vi "R4SetOtherConstants.vi"(6 "cRIONo":i32=1, 7 "LabVIEW Web Service Request":refnum<class "Web Request.lvclass">, 8 "ReactorNo":i32=1, 9 "Value":string, 10 "Constant":string, 11 "Write":bool) -> (1 "NewValue":string, 2 "OldValue":string, 3 "Status":string)   [LabVIEW 2016]
uses:
  <vilib>/wsapi/Web Request.lvclass
  <resource>/objmgr/ni.var.rc
panel:
  in  "LabVIEW Web Service Request 2":refnum<class "Web Request.lvclass">
  # "Use the Web Service Request input terminal to call the VIs on the Web Services palette. Do not remove it from the connector pane unless you don't need access to the palette."
  # "Each additional control wired to the connector pane will be available as an input in the URL. To include an indicator in terminal-mode output (the default setting), it must also be wired to the connector pane."
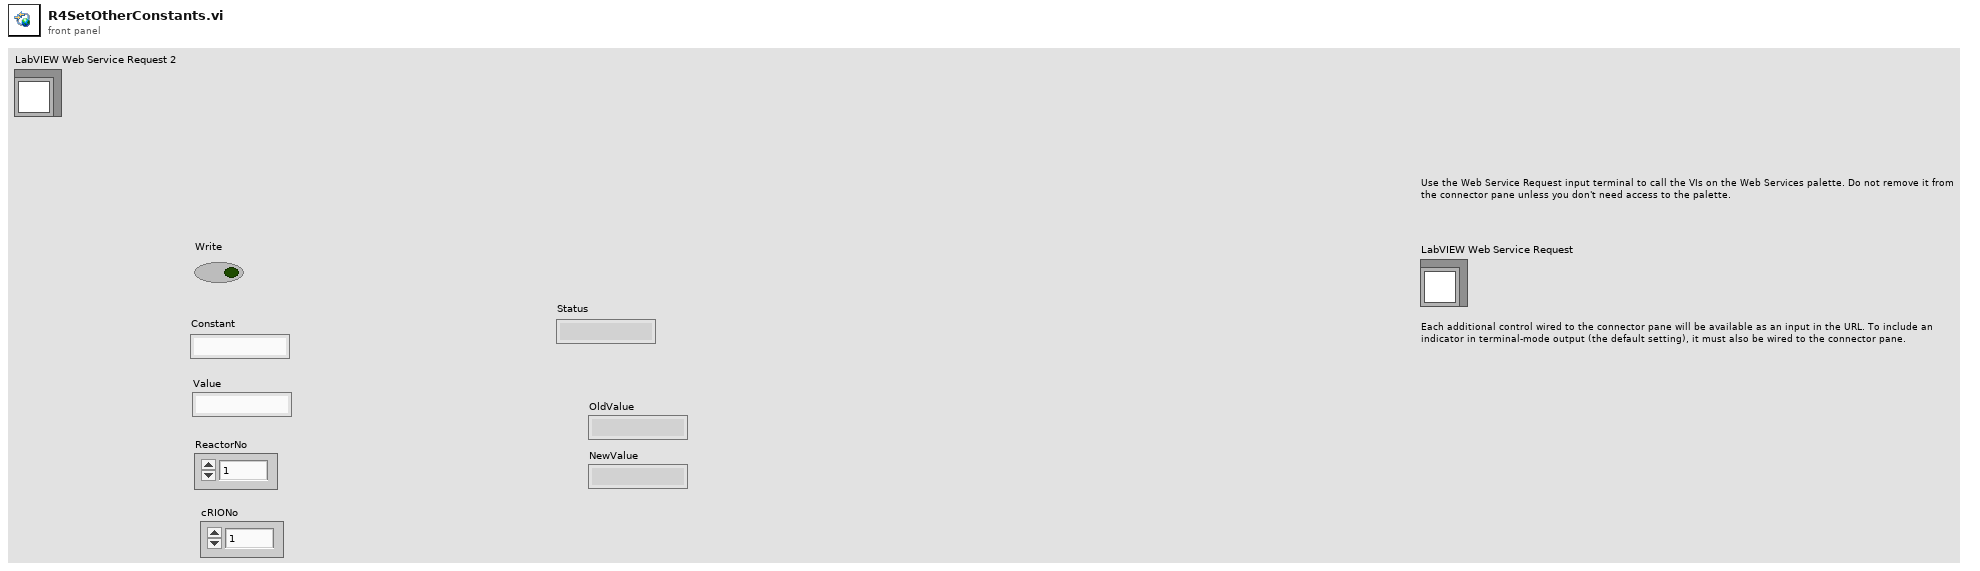
[diagram p1: front panel]
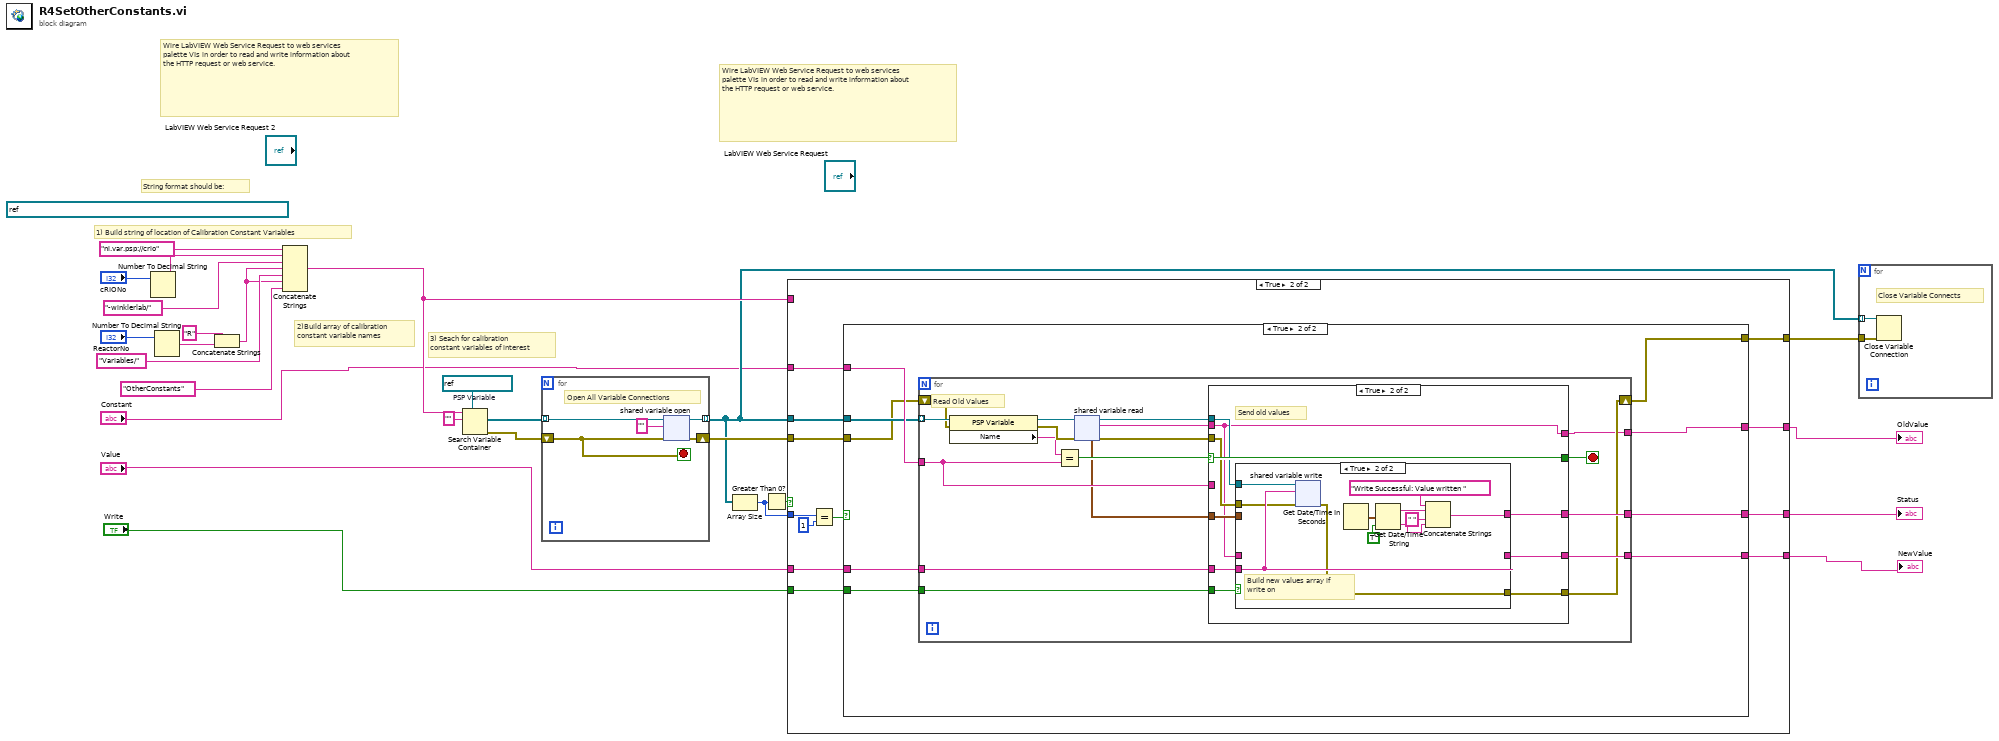
[diagram p0: block diagram]
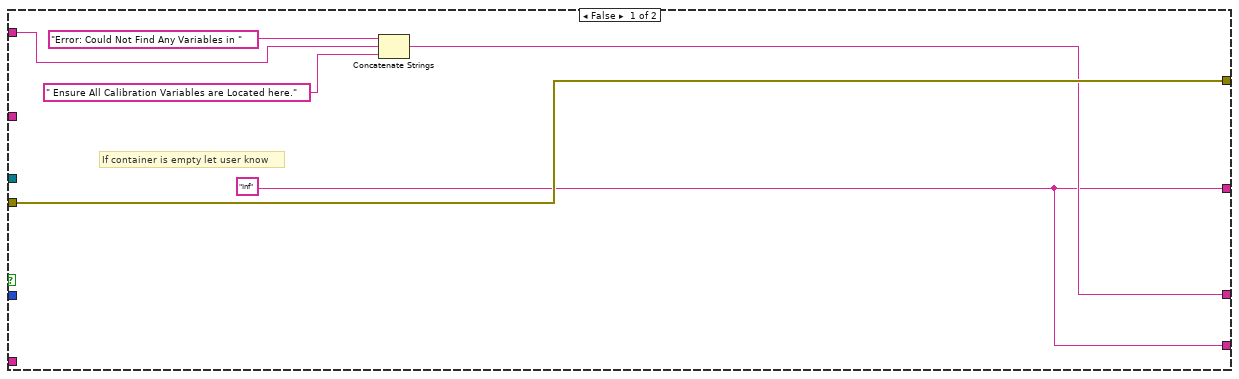
[diagram p2: hidden frame]
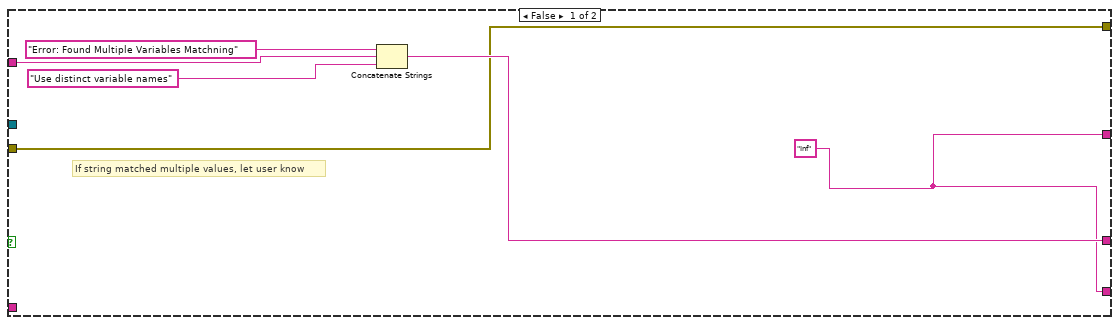
[diagram p3: hidden frame]
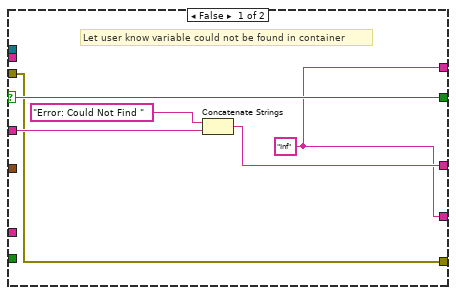
[diagram p4: hidden frame]
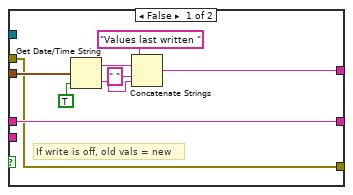
[diagram p5: hidden frame]
diagram:
  w16 = refnum<k21> refnum  # PSP Variable
  (unwired) refnum<k21> "ni.var.psp://crio1-winklerlab/R1Variables/R1OtherConstants" ("container refnum in")
  # "3) Seach for calibration \nconstant variables of interest"
  # "2)Build array of calibration \nconstant variable names"
  # "1) Build string of location of Calibration Constant Variables"
  # "String format should be:"
  # "Wire LabVIEW Web Service Request to web services palette VIs in order to read and write information about the HTTP request or web service."
  # "Wire LabVIEW Web Service Request to web services palette VIs in order to read and write information about the HTTP request or web service."
  n1 = Number To Decimal String(number="cRIONo") -> (decimal integer string=w21:string)  [unwired: 1 in]
  n2 = Number To Decimal String(number="ReactorNo") -> (decimal integer string=w24:string)  [unwired: 1 in]
  n3 = Concatenate Strings("R" ("string"), w24) -> (w18:string)
  n4 = Concatenate Strings("ni.var.psp://crio" ("string"), w21, "-winklerlab/" ("string"), w18, "Variables/" ("string"), w18, "OtherConstants" ("string")) -> (w10:string)
  n5 = Search Variable Container(7:w16, 10:"" ("regular expression"), 11:w10) -> (0:w13:errorcluster, 2:w14:refnum<k21>[])  [unwired: 3 in, 1 out]
  n6 = for {
    tunnel: w14 -> [w28] mode=indexing
    shift-right: [w31] -> w12
    shift-left: w13 -> [w29]
    tunnel: [w30] -> w7 mode=indexing
    stop <- w29 stop-if-true
    # "Open All Variable Connections"
    n7 = shared-variable-open(w28, w29, "" ("regular expression")) -> (w30:refnum<k21>, w31:errorcluster)  [unwired: 1 in]
  }
  n8 = Array Size(array=w7) -> (size(s)=w9:i32)
  n9 = Greater Than 0?(x=w9) -> (x > 0?=w11:bool)
  n10 = case shown="True" w11 {
    tunnel: "Constant" -> [_ w49]
    tunnel: "Write" -> [_ w48]
    tunnel: w7 -> [_ w47]
    tunnel: w12 -> [w34 w46]
    tunnel: w10 -> [w36 _]
    tunnel: w9 -> [_ w43]
    tunnel: [w34 w42] -> w8
    tunnel: [w32 w38] -> w3
    tunnel: [w32 w39] -> w4
    tunnel: [w33 w41] -> w6
    tunnel: "Value" -> [_ w40]
    frame False {
      w32 = "Inf"
      # "If container is empty let user know"
      n11 = Concatenate Strings("Error: Could Not Find Any Variables in " ("string"), w36, " Ensure All Calibration Variables are Located here." ("string")) -> (w33:string)
    }
    frame True {
      n12 = Equal?(x=w43, y=1) -> (x = y?=w45:bool)
      n13 = case shown="True" w45 {
        tunnel: w49 -> [w53 w64]
        tunnel: w48 -> [_ w63]
        tunnel: w40 -> [_ w62]
        tunnel: [w52 w61] -> w41
        tunnel: w47 -> [_ w60]
        tunnel: w46 -> [w51 w59]
        tunnel: [w51 w58] -> w42
        tunnel: [w50 w57] -> w39
        tunnel: [w50 w56] -> w38
        frame False {
          w50 = "Inf"
          # "If string matched multiple values, let user know"
          n14 = Concatenate Strings("Error: Found Multiple Variables Matchning" ("string"), w53, "Use distinct variable names" ("string")) -> (w52:string)
        }
        frame True {
          n15 = for {
            tunnel: w60 -> [w73] mode=indexing
            tunnel: w64 -> [w75]
            tunnel: w63 -> [w78]
            tunnel: [w67] -> w57
            tunnel: [w77] -> w56
            tunnel: [w76] -> w61
            tunnel: w62 -> [w65]
            shift-right: [w68] -> w58
            shift-left: w59 -> [w71]
            stop <- w74 stop-if-true
            # "Read Old Values"
            n16 = property class="PSP Variable"(reference=w73, error in=w71) -> (reference out=w72:refnum<k21>, error out=w70:errorcluster, "Name"=w69:string)
            n17 = Equal?(x=w69, y=w75) -> (x = y?=w79:bool)
            n18 = shared-variable-read(w72, w70) -> (w82:refnum<k21>, w80:errorcluster, w81:string, w66:timestamp)
            n19 = case shown="True" w79 {
              selector: w79 -> [w88 w98]
              tunnel: w82 -> [_ w93]
              tunnel: w81 -> [_ w90]
              tunnel: w80 -> [w84 w92]
              tunnel: [w88 w98] -> w74
              tunnel: [w83 w90] -> w67
              tunnel: w66 -> [_ w97]
              tunnel: w78 -> [_ w96]
              tunnel: [w83 w89] -> w77
              tunnel: [w85 w95] -> w76
              tunnel: w75 -> [w86 _]
              tunnel: w65 -> [_ w94]
              tunnel: [w84 w91] -> w68
              frame False {
                w83 = "Inf" ("string")
                # "Let user know variable could not be found in container"
                n20 = Concatenate Strings("Error: Could Not Find " ("string"), w86) -> (w85:string)
              }
              frame True {
                # "Send old values"
                n21 = case shown="True" w96 {
                  tunnel: w97 -> [w106 _]
                  tunnel: [w102 w112] -> w95
                  tunnel: w90 -> [w100 _]
                  tunnel: [w100 w110] -> w89
                  tunnel: w94 -> [_ w110]
                  tunnel: w93 -> [_ w111]
                  tunnel: w92 -> [w99 w109]
                  tunnel: [w99 w108] -> w91
                  frame False {
                    # "If write is off, old vals = new"
                    n22 = Get Date/Time String(seconds (now)=w106, want seconds? (F)=TRUE) -> (date string=w105:string, time string=w103:string)  [unwired: 1 in]
                    n23 = Concatenate Strings("Values last written " ("string"), w105, " " ("string"), w103) -> (w102:string)
                  }
                  frame True {
                    # "Build new values array if \nwrite on"
                    n24 = shared-variable-write(w111, w109, w110) -> (w108:errorcluster)  [unwired: 1 out]
                    n25 = Get Date/Time In Seconds() -> (seconds since 1Jan1904=w113:timestamp)
                    n26 = Get Date/Time String(seconds (now)=w113, want seconds? (F)=TRUE) -> (date string=w115:string, time string=w117:string)  [unwired: 1 in]
                    n27 = Concatenate Strings("Write Successful: Value written " ("string"), w115, " " ("string"), w117) -> (w112:string)
                  }
                }
              }
            }
          }
        }
      }
    }
  }
  "OldValue" <- w4
  "NewValue" <- w3
  "Status" <- w6
  n28 = for {
    tunnel: w8 -> [w119]
    tunnel: w7 -> [w120] mode=indexing
    # "Close Variable Connects"
    n29 = Close Variable Connection(8:w119, 11:w120) -> ()  [unwired: 1 out]
  }
